vi "Eye Movement Analyser.vi"(7 "Data Output":T12 {"Data Channels" format="%.2f"}) -> ()   [LabVIEW 2016]
uses:
  core/type-defs/TD_Time Series.ctl
  core/type-defs/TD_Impulse Parameter.ctl
  core/private/Impulse Analyser state.ctl
  core/type-defs/TD_Event Sequencer.ctl
  <vilib>/Utility/miscctls.llb/LVRowAndColumnUnsignedTypeDef.ctl
  <vilib>/Analysis/baseanly.llb/Unit Vector (DBL).vi
  <vilib>/Analysis/1siggen.llb/Ramp Pattern by Samples.vi
  <vilib>/Analysis/baseanly.llb/Real Dot Product.vi
  <vilib>/Analysis/baseanly.llb/Mean (DBL).vi
  <vilib>/Utility/inputDevices.llb/mouseAcquire.vi
  <userlib>/_OpenG.lib/comparison/comparison.llb/Boolean Changed__ogtk.vi
  plugins/Mars 3D/Mars3D_autosort.vi
  <vilib>/Utility/file.llb/Read From Spreadsheet File (DBL).vi
  <userlib>/_OpenG.lib/file/file.llb/File Exists - Scalar__ogtk.vi
  <userlib>/_OpenG.lib/array/array.llb/Sort 1D Array (I32)__ogtk.vi
  core/Classes/Graph Manager/Graph Manager.lvclass
  comm/impulse/impulse functions.lvlib
  comm/comm.lvlib
  plugins/Report/generate report.lvlib
  comm/quaternion/quaternion.lvlib
  comm/fick-matrix/fick-matrix.lvlib
  <vilib>/Analysis/NI_AALBase.lvlib
  <vilib>/Analysis/NI_AALPro.lvlib
  <vilib>/Analysis/baseanly.llb/A x Vector.vi
  core/core.lvlib
  comm/double click/double click.lvlib
  plugins/plugin data.lvlib
  <vilib>/ptbypt/NI_PtbyPt.lvlib
  comm/nan operations/nan operations.lvlib
panel:
  out "Time series Trace":cluster{dbl, dbl, dbl[][]}(graph) caption="Waveform Graph"
  in  "Tab Control":T1(tab)
  in  "EyeSeeCam":bool
  in  "Chair":bool
  in  "Mars Training":bool
  in  "3D Chincilla":bool
  in  "Mars 3D 2":bool
  in  "Mars 3D":bool
  in  "JHOC":bool
  in  "Load Data":bool
  in  "Wireless":bool
  in  "Append Data":bool
  in  "Btn Clear Temp LVS":bool
  in  "Update Batch File":bool
  in  "Load Batch File":bool
  in  "Batch Next":bool
  in  "Experiment Files":i32(listbox)
  in  "Parameter Time Series":T2 {"time offset" format="%.3f"; "Gain" format="%.1f"; "Offset" format="%.1f"; "List 1" items=["Hz Position-in-Head", "Hz Velocity-in-Head", "Hy Position-in-Head", "Hy Velocity-in-Head", "Hx Position-in-Head", "Hx Velocity-in-Head", "Hl Velocity-in-Head", "Hr Velocity-in-Head", "Lx Position-in-Head", "Ly Position-in-Head", "Lz Position-in-Head", "Lx Velocity-in-Head", "Ly Velocity-in-Head", "Lz Velocity-in-Head", "Ll Velocity-in-Head", "Lr Velocity-in-Head", "Rx Position-in-Head", "Ry Position-in-Head", "Rz Position-in-Head", "Rx Velocity-in-Head", "Ry Velocity-in-Head", "Rz Velocity-in-Head", "Rl Velocity-in-Head", "Rr Velocity-in-Head", "Target on/off", "aux input 1", "aux input 2", " ", "", "", "", "Target Hor", "Target Ver", ""]}
  in  "Filter Method":u16(ring)=1 items=["Savitzky Golay", "FIR Filter", "Spline"]
  out "Tab Control 2":enum32{"Page 2", "Page 3", "Page 1"}(tab)=enum."Page 3"
  in  "Filter characteristics":T3={"Filter type"=enum."Lowpass", "Order"=50, "Higher pass freq"=40.0, "Lower pass freq"=40.0} {"Lower pass freq" format="%.2f"; "Higher pass freq" format="%.2f"}
  in  "Filter Data":bool
  in  "Gl Spline":bool caption="Enable Spline for all Channels"
  out "R-sq":dbl
  in  "Spline balance parameter":dbl=0.9 min=0.9 max=1.0 step=1e-07 format="%#_7g"
  in  "spline":bool
  in  "Interpolate":bool=TRUE
  in  "S-pline":bool
  out "calibration filename":string
  out "filename":string
  in  "Fixed Time 2":bool caption="Fixed Time"
  in  "Fixed Amplitude 2":bool caption="Fixed Amplitude"
  out "dY":dbl format="%#12.3f"
  out "dX":dbl format="%#10.1f"
  in  "Time Cursor Color 2":u32(colorbox)=16711680
  in  "Time Curser Y2":dbl caption="Y:" format="%_4g"
  in  "Time Curser X2":dbl caption="X:" format="%_4g"
  in  "Time Cursor Color 1":u32(colorbox)=16711680
  in  "Time Curser Y1":dbl caption="Y:" format="%_4g"
  in  "Time Curser X1":dbl caption="X:" format="%_4g"
  in  "Cut":bool
  in  "Keep in range":bool
  in  "Generate New Plot":bool
  out "Impulse Trace":cluster{dbl, dbl, "Impulses":dbl[][]}(graph)
  in  "Asymmetry Plot":bool
  in  "Main Sequence Saccade":bool
  in  "Time Constant Plugin":bool
  in  "Reset to Raw":bool
  in  "Analyze Saccades":bool
  in  "Autosort Name":string
  in  "Auto Sort Parameter":u16(ring) items=["xxx"]
  in  "Impulse Analyser":bool
  in  "Gain and Phase":bool
  in  "Dots":bool
  in  "off and gains perm":bool
  in  "Saccade Velocity":bool
  in  "De-Saccading":bool
  in  "Impulse Parameters":bool
  in  "Group Analyser":bool
  in  "Threshold 2 [% of TH-1]":i32(slide) scale=0.0..100.0
  in  "Tolerance [ms]":dbl(slide)=39.7 step=0.1 scale=0.0..100.0
  in  "Tab Control 3":T4(tab)
  in  "Eye Movement Analyser":bool
  in  "Trigger Method":T5(ring)
  in  "Impulse surround":T6={"Pre Impulse (ms)"=150, "Post Impulse (ms)"=150, "LARP / RALP trigger Vel"=15.0} {"LARP / RALP trigger Vel" format="%.2f"}
  in  "Impulse Characteristics":T7={"Min Vel /Trigger"=90.0, "Width / Offset (ms)"=100, "Maximum Velocity"=300.0} {"Maximum Velocity" format="%.2f"; "Min Vel /Trigger" format="%.2f"}
  in  "Impulse Plane":bool
  in  "Trigger Channel (Other)":u16(ring)=1 items=["Hz Position-in-Head", "Hz Velocity-in-Head", "Hy Position-in-Head", "Hy Velocity-in-Head", "Hx Position-in-Head", "Hx Velocity-in-Head", "Hl Velocity-in-Head", "Hr Velocity-in-Head", "Lx Position-in-Head", "Ly Position-in-Head", "Lz Position-in-Head", "Lx Velocity-in-Head", "Ly Velocity-in-Head", "Lz Velocity-in-Head", "Ll Velocity-in-Head", "Lr Velocity-in-Head", "Rx Position-in-Head", "Ry Position-in-Head", "Rz Position-in-Head", "Rx Velocity-in-Head", "Ry Velocity-in-Head", "Rz Velocity-in-Head", "Rl Velocity-in-Head", "Rr Velocity-in-Head", "Target on/off", "aux input 1", "aux input 2", " ", "", "", "", "Target Hor", "Target Ver", ""]
  in  "Del Autosort":bool
  in  "Add Autosort":bool
  in  "Cross Correlation":bool
  in  "Impulse Characteristic from Cursor":bool caption="Select one periode of the signal"
  in  "Default":bool
  in  "Add Autosort OK":bool
  in  "Add Autosort Cancel":bool
  in  "Accel Threshold [TH-1]":dbl(slide)=3000.0 step=10.0 scale=100.0..1000000.0
  in  "Velocity Threshold":i32(slide)=203 scale=0.0..400.0
  in  "SD for Outlier detection":dbl(slide) scale=0.0..5.0
  in  "Live Update":bool=TRUE
  in  "Reset To default":bool
  in  "Search Window [ms]":i32(slide)=151 scale=0.0..500.0
  in  "Capture Saccade":bool=TRUE
  in  "Display Saccade":bool
  in  "Saccade width [ms]":cluster{i32, i32}(slide)={0, 3} scale=0.0..400.0
  out "Fits a line to a noisy slow-phase. First 3 channels in plot window (above) must be x, y, and z eye position in that order.":dbl[][](graph)
  in  "Sac Vel":bool
  out "HOR\n\nLARP\n\nRALP":dbl[](array[numeric]) format="%#_2g"
  out "X deg/s      Y deg/s      Z deg/s":dbl[](array[numeric]) format="%#_3g"
  out "Mean Ch 1":dbl
  out "Mean Ch2":dbl
  out "Mean Ch3":dbl
  in  "Only Use TH-2":bool
  out "Other Trigger channel":bool
  in  "Shortcut 3":bool
  in  "Shortcut 2":bool
  in  "Shortcut 1":bool
  out "Acc":dbl
  out "Vel.":dbl
  out "Freq.":dbl
  out "Stimulus type":string
  out "No. Imp":i32 caption="# Imp"
  in  "Help":bool
  in  "Options":bool
  in  "Save Image Impulse":bool
  in  "Export TS":bool
  in  "Save Data":bool
  in  "Export Data":bool
  in  "Generate Report":bool
  in  "Redo":bool
  in  "Undo Last":bool
  in  "Undo Last 2":bool
  in  "Tab Control Impuls":enum32{"Page 1", "Page 3", "Page 2"}(tab)
  in  "Parameter Impuls Series":T8 caption="Offset    Gain       Inv                      Channel                            Vis   Sac" {"Gain" format="%.1f"; "Offset" format="%.1f"; "Channel" items=["Hz Position-in-Head", "Hz Velocity-in-Head", "Hy Position-in-Head", "Hy Velocity-in-Head", "Hx Position-in-Head", "Hx Velocity-in-Head", "Hl Velocity-in-Head", "Hr Velocity-in-Head", "Lx Position-in-Head", "Ly Position-in-Head", "Lz Position-in-Head", "Lx Velocity-in-Head", "Ly Velocity-in-Head", "Lz Velocity-in-Head", "Ll Velocity-in-Head", "Lr Velocity-in-Head", "Rx Position-in-Head", "Ry Position-in-Head", "Rz Position-in-Head", "Rx Velocity-in-Head", "Ry Velocity-in-Head", "Rz Velocity-in-Head", "Rl Velocity-in-Head", "Rr Velocity-in-Head", "Target on/off", "aux input 1", "aux input 2", " ", "", "", "", "Target Hor", "Target Ver", ""]}
  in  "Generate New Impulse Plot":bool
  in  "Mean and STD":bool
  in  "Impulse dir":bool
  in  "Impulse Plane 2":T9(ring)=enum."Yaw" caption="Plane"
  in  "Reset Save Options":bool
  in  "Aligning Channel":u16(ring)=5 items=["Hz Position-in-Head", "Hz Velocity-in-Head", "Hy Position-in-Head", "Hy Velocity-in-Head", "Hx Position-in-Head", "Hx Velocity-in-Head", "Hl Velocity-in-Head", "Hr Velocity-in-Head", "Lx Position-in-Head", "Ly Position-in-Head", "Lz Position-in-Head", "Lx Velocity-in-Head", "Ly Velocity-in-Head", "Lz Velocity-in-Head", "Ll Velocity-in-Head", "Lr Velocity-in-Head", "Rx Position-in-Head", "Ry Position-in-Head", "Rz Position-in-Head", "Rx Velocity-in-Head", "Ry Velocity-in-Head", "Rz Velocity-in-Head", "Rl Velocity-in-Head", "Rr Velocity-in-Head", "Target on/off", "aux input 1", "aux input 2", " ", "", "", "", "Target Hor", "Target Ver", ""]
  in  "Horizontal Align":bool
  in  "Vertical Align":bool
  in  "Acceleration":bool
  in  "Autosize Parameter Set":i8(ring) caption="Trigger Set" items=["No Set selected", "Mars 3D", "", "3D Chinchilla", "", "visStim", "", "", "", "", "Human Rotary Chair"]
  in  "Trace":i32 min=0 max=1000
  in  "Paint delete":bool=TRUE
  in  "Cut After":bool
  in  "Cut Before":bool
  in  "Fixed Time":bool
  in  "Fixed Amplitude":bool
  in  "Impuls Cursor Y":dbl caption="Y:"
  in  "Impuls Cursor X":dbl caption="X:"
  out "loaded filename":path
  in  "Head coord":bool
  in  "Target position":T10(ring)
  in  "H":dbl format="%.2f"
  in  "Change coord":bool
  in  "Old Impulse positions for Undo":T11(array[cluster]) {"Amplitude offset" format="%.2f"}
  in  "Impulse Positions":T11(array[cluster]) {"Amplitude offset" format="%.2f"}
  out "axis info":T13
  in  "Delete Impulse":bool
  out "LVS data path":path=path "/Macintosh HD/Users/patrick/Studium/Diploma Thesis/Data Analysis"
  in  "Stop":bool
  in  "Human VOG":bool
  in  "galvanic":bool
  in  "COR":bool
  in  "T":dbl format="%.2f"
  in  "V":dbl format="%.2f"
  in  "Optotrak":bool
  in  "Finnish":bool
  in  "NTA":bool
  in  "ASCII":bool
  in  "Process Coils Data 2":bool
  in  "Process Animal Data":bool
  in  "Process Coils Data":bool
  out "Processing":bool
  # "Description"
  # "<-- Belongs Here"
  # "Rarely used buttons"
  # "FOR COORD\nCHANGE ORDER IS\nXvel,\nYvel,\nZvel,\nLvel,\nRvel"
  # "Cursor:"
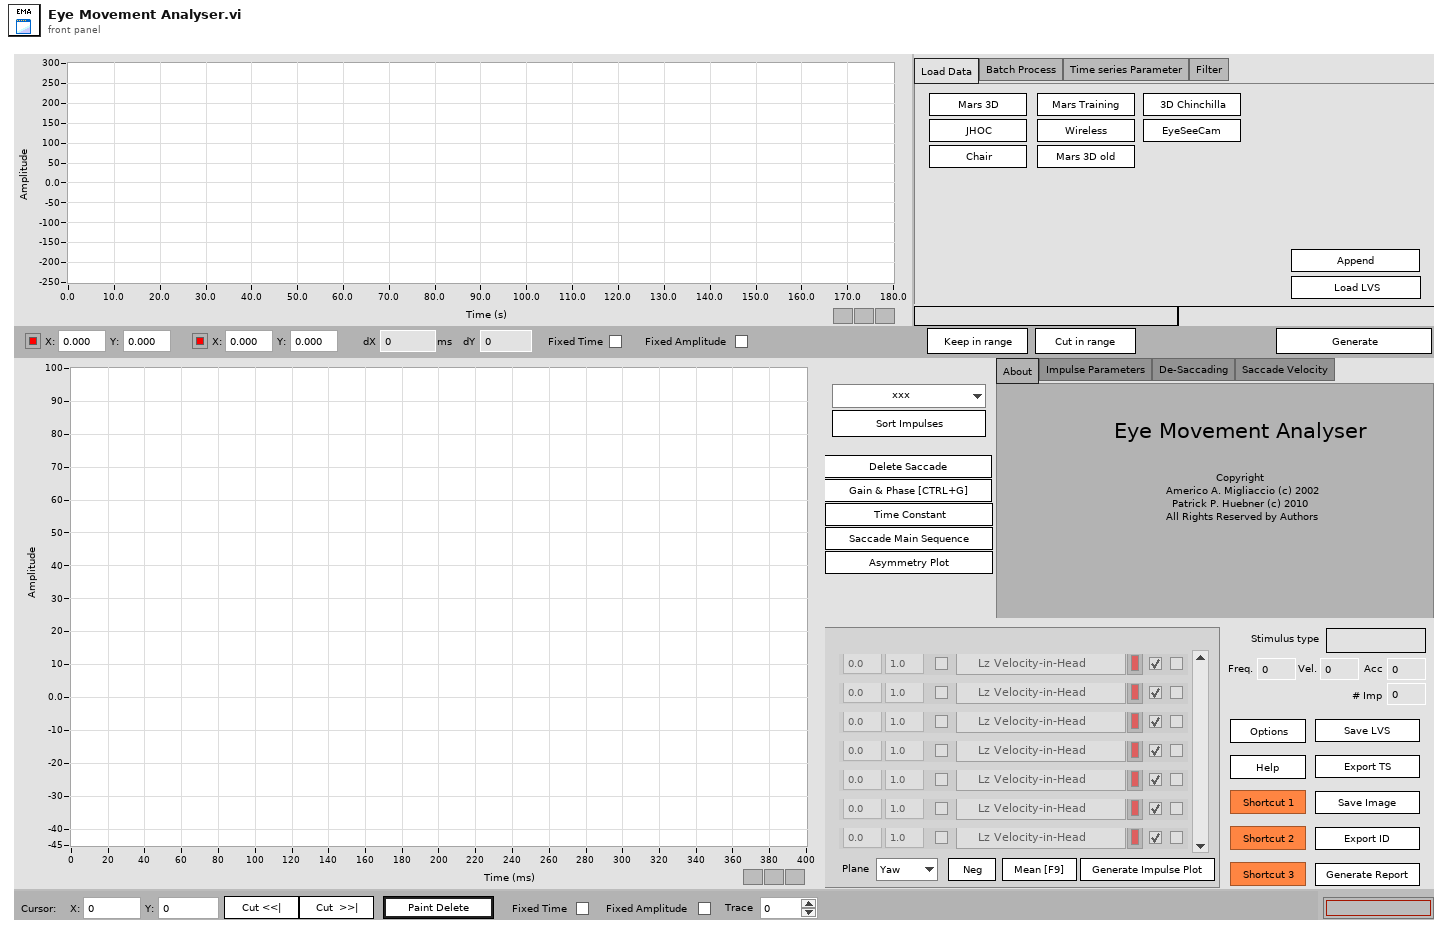
[diagram p1: front panel]
types:
  T1 = enum32{"Load Data", "Batch Process", "Time series Parameter", "Filter"}
  T2 = typedef "core.lvlib/TD_Time Series.ctl" = cluster{"time offset":dbl, "Offset":dbl, "Gain":dbl, "inverse":bool, "filter data":bool, "dots":bool, "interpolate":bool, "List 1":u16, "Color Box":u32, "Boolean":bool}[]
  T3 = cluster{"Filter type":enum32{"Lowpass", "Highpass", "Bandpass", "Bandstop"}, "Order":i32, "Higher pass freq":dbl, "Lower pass freq":dbl}
  T4 = enum32{"About", "Impulse Parameters", "De-Saccading", "Saccade Velocity"}
  T5 = enum16{"Peak Detektion", "Rising Edge", "Falling Edge", "Rising Edge (multiple)", "Falling Edge (multiple)"}
  T6 = cluster{"Pre Impulse (ms)":i32, "Post Impulse (ms)":i32, "LARP / RALP trigger Vel":dbl}
  T7 = cluster{"Min Vel /Trigger":dbl, "Width / Offset (ms)":i32, "Maximum Velocity":dbl}
  T8 = typedef "core.lvlib/TD_Impulse Parameter.ctl" = cluster{"Color":u32, "Visible":bool, "Channel":u16, "Invert":bool, "Desaccade":bool, "Offset":dbl, "Gain":dbl}[]
  T9 = enum16{"Other", "Yaw", "Pitch", "Roll", "LARP", "RALP"}
  T10 = enum16{"Far 0", "Far Left 20", "Far Left 30", "Far right 30", "Far Right 20", "Near 0", "Near Left 20", "Near Right 20"}
  T11 = cluster{"Start":i32, "End":i32, "Impulse Plane":enum16{"Other", "Yaw", "Pitch", "Roll", "LARP", "RALP"}, "Impulse Direction +ve?":bool, "Time offset":i32, "Amplitude offset":dbl}[]
  T12 = cluster{"Data Channels":dbl[][], "Sample Rate":i32, "Channel List":string[]}
  T13 = cluster{"Horizontal":i32, "Vertical":i32, "Scrolling":i32}
  T14 = typedef "Impulse Analyser state.ctl" = enum16{"--- System ---", "Panel Monitoring", "Check Save Status", "Initialize", "Initialise GUI", "Quit", "--- Import ---", "Desaccade Time Data", "Desaccade Time Data Background", "Paint Delete", "Load Batch Log File", "Make Batch List", "Update Batch List", "Delete Batch List", "Delete Temporary LVS", "Save Temporary LVS", "Check for Batch LVS", "Process 3D Chinchilla", "Find default parameter", "Mars3D old", "Chair", "EyeSeeCam", "Open last session", "Save RAW", "Auto Impulse Parameter", "Save Image", "Wireless", "Process Coils Data", "Process JHOC Data", "Process Animal Data", "Australian Data", "ASCII", "Mars 3D", "Mars 3D Training", "Position Mean Plugin", "plot generator plugin", "Human VOG system", "Optotrak", "spline", "COR", "galvanic", "Generate New Time Plot", "Make off and gains permanent", "Generate New Impulse Plot", "Defer Impulse Plot", "Fill Impulse Plot Data", "Scale Impulse Plot", "Un-Defer Impulse Plot", "Snap Impulse Cursor", "Extract Saccades", "Impulse Analyser", "NTA", "Acceleration", "Saccade Velocity", "Horizontal Align", "Vertical Align", "Delete Impulse", "Cut Before", "Cut After", "Filter Data", "Undo Last", "Redo", "Mean and STD", "Group Analyser", "Generate Report", "Phase Plots", "Gain and Phase", "Example Plugin", "Time Constant Plugin", "Export Data", "Export Time Series Data", "Append Data", "Save Data", "Load Data", "Cut in Range", "Keep in range", "Stop"}
  T15 = typedef "TD_Event Sequencer.ctl" = enum16{"Core", "Plugins"}
  T16 = enum8{"Enabled", "Disabled", "Disabled and Grayed Out"}
  T17 = cluster{"Save RAW":bool, "Save Options":bool, "Save IMAGE":bool, "Cycle Nr for Saccades":cluster{"POS":i32, "NEG":i32}, "Paint Delete":bool, "device ID":refnum<k1>, "Delete-Array":i32[], "Double Click":refnum<event-registration>, "DC file":path, "Session saved?":bool}
  T18 = cluster{"Start":i32, "End":i32, "Impulse Plane":enum16{"Other", "Yaw", "Pitch", "Roll", "LARP", "RALP"}, "Impulse Direction +ve?":bool, "Time offset":i32, "Amplitude offset":dbl}
  T19 = enum16{"open", "open or create", "create or replace", "create", "open (read only)"}
  T20 = typedef "LVRowAndColumnUnsignedTypeDef.ctl" = cluster{"Row":u32, "Column":u32}
  T21 = enum16{"open", "replace", "create", "open or create", "replace or create", "replace or create with confirmation"}
  T22 = enum16{"Left Button", "Center Button", "Right Button", "Window Close"}
  T23 = cluster{"Impulse Positions":cluster{"Start":i32, "End":i32, "Impulse Plane":enum16{"Other", "Yaw", "Pitch", "Roll", "LARP", "RALP"}, "Impulse Direction +ve?":bool, "Time offset":i32, "Amplitude offset":dbl}[], "Old Impulse positions for Undo":cluster{"Start":i32, "End":i32, "Impulse Plane":enum16{"Other", "Yaw", "Pitch", "Roll", "LARP", "RALP"}, "Impulse Direction +ve?":bool, "Time offset":i32, "Amplitude offset":dbl}[], "No. Imp":i32, "Parameter Time Series":T2, "Parameter Impuls Series":T8, "Experiment Parameters":cluster{"Freq":dbl, "Vel":i32, "Acc":i32, "Stimulus":string}, "Autosort File":refnum<file>, "Data File":cluster{"Data Channels":dbl[][], "Sample Rate":i32, "Channel List":string[]}, "Experiment data path":path, "Image data path":path, "LVS data path":path, "Raw copy path":path, "filename":string, "desaccading parameters":cluster{"Tolerance":i32, "Acc Range":dbl, "Sample Rate":i32, "Impulse Plane 2":enum16{"Other", "Yaw", "Pitch", "Roll", "LARP", "RALP"}, "Impulse dir":bool}, "Experiment Parameters 2":cluster{"Subject":string, "Strain":string, "Rotation plane":string, "Experimenter":string, "Trial":dbl, "Time":dbl}, "Excel":cluster{"Excel._Application":refnum<k7>, "Use Excel":bool, "Worksheet SINE":refnum<k7>, "Row SINE":i32, "Worksheet TRANS":refnum<k7>, "Row TRANS":i32}, "Session Config File":refnum<file>, "Autosort Parameter Set":i32, "EMA Version":string, "desacc ":cluster{"Threshold 1 [Acc]":dbl, "Threshold 2 [% of TH1]":i32, "tolerance":i32, "Search WD ":dbl, " always use TH2":bool, "Range":dbl, "Max time":dbl, "Min time":dbl}}
  T24 = cluster{"Subject":string, "Strain":string, "Rotation plane":string, "Experimenter":string, "Trial":dbl, "Time":dbl}
  T25 = cluster{"Freq":dbl, "Vel":i32, "Acc":i32, "Stimulus":string}
  T26 = cluster{"Impulse Positions":cluster{"Start":i32, "End":i32, "Impulse Plane":enum16{"Other", "Yaw", "Pitch", "Roll", "LARP", "RALP"}, "Impulse Direction +ve?":bool, "Time offset":i32, "Amplitude offset":dbl}[], "Old Impulse positions for Undo":cluster{"Start":i32, "End":i32, "Impulse Plane":enum16{"Other", "Yaw", "Pitch", "Roll", "LARP", "RALP"}, "Impulse Direction +ve?":bool, "Time offset":i32, "Amplitude offset":dbl}[], "No. Imp":i32}
  T27 = typedef "LVPoint32TypeDef.ctl" = cluster{"Horizontal":i32, "Vertical":i32}
  T28 = cluster{"button 1":bool, "button 2":bool, "button 3":bool, "button 4":bool}
  T29 = cluster{"Fixed Time":bool, "Fixed Amplitude":bool}
  T30 = typedef "core.lvlib/TD_Statemachine-Data.ctl" = cluster{"Impulse Positions":cluster{"Start":i32, "End":i32, "Impulse Plane":enum16{"Other", "Yaw", "Pitch", "Roll", "LARP", "RALP"}, "Impulse Direction +ve?":bool, "Time offset":i32, "Amplitude offset":dbl}[], "Old Impulse positions for Undo":cluster{"Start":i32, "End":i32, "Impulse Plane":enum16{"Other", "Yaw", "Pitch", "Roll", "LARP", "RALP"}, "Impulse Direction +ve?":bool, "Time offset":i32, "Amplitude offset":dbl}[][], "No. Imp":i32, "Parameter Time Series":T2, "Parameter Impuls Series":T8, "Experiment Parameters":cluster{"Freq":dbl, "Vel":i32, "Acc":i32, "Stimulus":string}, "Autosort File":refnum<file>, "Data File":cluster{"Data Channels":dbl[][], "Sample Rate":i32, "Channel List":string[]}, "Experiment data path":path, "Image data path":path, "LVS data path":path, "Raw copy path":path, "filename":string, "desaccading parameters":cluster{"Tolerance":i32, "Acc Range":dbl, "Sample Rate":i32, "Impulse Plane 2":enum16{"Other", "Yaw", "Pitch", "Roll", "LARP", "RALP"}, "Impulse dir":bool}, "Experiment Parameters 2":cluster{"Subject":string, "Strain":string, "Rotation plane":string, "Experimenter":string, "Trial":dbl, "Time":dbl}, "Excel":cluster{"Excel._Application":refnum<k7>, "Use Excel":bool, "Worksheet SINE":refnum<k7>, "Row SINE":i32, "Worksheet TRANS":refnum<k7>, "Row TRANS":i32}, "Session Config File":refnum<file>, "Autosort Parameter Set":i32, "EMA Version":string, "desacc ":cluster{"Threshold 1 [Acc]":dbl, "Threshold 2 [% of TH1]":i32, "tolerance":i32, "Search WD ":dbl, " always use TH2":bool, "Range":dbl, "Max time":dbl, "Min time":dbl, "Velocity Threshold":i32}, "Cycle Nr for Saccades":cluster{"POS":i32, "NEG":i32}, "Undo Counter":i32, "History Length":i32, "Redo Counter":i32, "Histpry Position":i32, "Raw Data File":cluster{"Data Channels":dbl[][], "Sample Rate":i32, "Channel List":string[]}, "calibration name":string}
  T31 = cluster{"Threshold 1 [Acc]":dbl, "Threshold 2 [% of TH1]":i32, "tolerance":i32, "Search WD ":dbl, " always use TH2":bool, "Range":dbl, "Max time":dbl, "Min time":dbl, "Velocity Threshold":i32}
  T32 = cluster{"Tolerance [ms]":dbl, "Accel Threshold [TH-1]":dbl, "Sample Rate":i32, "Impulse Plane 2":enum16{"Other", "Yaw", "Pitch", "Roll", "LARP", "RALP"}, "Impulse dir":bool}
  T33 = typedef "eventvkey.ctl" = enum16{"ASCII", "Enter", "Return", "Shift", "Ctrl", "Alt", "Cmd", "Opt", "Caps", "NumLock", "Clear", "Break", "Up", "Down", "Left", "Right", "Insert", "Delete", "Home", "End", "PageUp", "PageDown", "Escape", "Help", "Pause", "ScrollLock", "F1", "F2", "F3", "F4", "F5", "F6", "F7", "F8", "F9", "F10", "F11", "F12", "F13", "F14", "F15", "F16", "F17", "F18", "F19", "F20", "F21", "F22", "F23", "F24", "Play", "VolumeUp", "VolumeDown", "Mute", "Two Byte Char"}
  T34 = cluster{"Shift":bool, "Ctrl":bool, "Alt":bool, "Cmd":bool, "Opt":bool}
  T35 = cluster{"Start":i32, "End":i32, "Impulse Plane":enum16{"Other", "Yaw", "Pitch", "Roll", "LARP", "RALP"}, "Impulse Direction +ve?":bool, "Time offset":i32, "Amplitude offset":dbl}[][]
  T36 = enum32{"invalid app kind", "Development System", "Run Time System", "Student Edition", "Embedded LabVIEW", "Evaluation", "Custom"}
  T37 = cluster{"Tolerance":i32, "Acc Range":dbl, "Sample Rate":i32, "Impulse Plane 2":enum16{"Other", "Yaw", "Pitch", "Roll", "LARP", "RALP"}, "Impulse dir":bool}
  T38 = cluster{"Impulse Positions":cluster{"Start":i32, "End":i32, "Impulse Plane":enum16{"Other", "Yaw", "Pitch", "Roll", "LARP", "RALP"}, "Impulse Direction +ve?":bool, "Time offset":i32, "Amplitude offset":dbl}[], "Old Impulse positions for Undo":cluster{"Start":i32, "End":i32, "Impulse Plane":enum16{"Other", "Yaw", "Pitch", "Roll", "LARP", "RALP"}, "Impulse Direction +ve?":bool, "Time offset":i32, "Amplitude offset":dbl}[][], "No. Imp":i32, "Parameter Time Series":T2, "Parameter Impuls Series":T8, "Experiment Parameters":cluster{"Freq":dbl, "Vel":i32, "Acc":i32, "Stimulus":string}, "Data File":cluster{"Data Channels":dbl[][], "Sample Rate":i32, "Channel List":string[]}, "Experiment data path":path, "Image data path":path, "LVS data path":path, "Raw copy path":path, "filename":string, "desaccading parameters":cluster{"Tolerance":i32, "Acc Range":dbl, "Sample Rate":i32, "Impulse Plane 2":enum16{"Other", "Yaw", "Pitch", "Roll", "LARP", "RALP"}, "Impulse dir":bool}, "Experiment Parameters 2":cluster{"Subject":string, "Strain":string, "Rotation plane":string, "Experimenter":string, "Trial":dbl, "Time":dbl}, "Autosort Parameter Set":i32, "calibration name":string}
  T39 = cluster{"Data Output":cluster{"Data Channels":dbl[][], "Sample Rate":i32, "Channel List":string[]}, "Data OUT":T30}
  T40 = cluster{"Autosize Parameter Set 2":cluster{"Trigger Ch":i32, "Min Vel":dbl, "MaxVel":dbl, "Width":i32, "Pre Impuls":i32, "Post Impuls":i32, "Pitch":dbl, "Name":string, "Other Trigger":bool, "Cross Corr":bool, "Default":cluster{"Freq":dbl, "Vel":dbl, "Acc":dbl, "Stimulus":string}}[]}[]
  T41 = cluster{"Autosize Parameter Set 2":cluster{"Trigger Ch":i32, "Min Vel":dbl, "MaxVel":dbl, "Width":i32, "Pre Impuls":i32, "Post Impuls":i32, "Pitch":dbl, "Name":string, "Other Trigger":bool, "Cross Corr":bool, "Default":cluster{"Freq":dbl, "Vel":dbl, "Acc":dbl, "Stimulus":string}}[]}
  T42 = cluster{"Trigger Ch":i32, "Min Vel":dbl, "MaxVel":dbl, "Width":i32, "Pre Impuls":i32, "Post Impuls":i32, "Pitch":dbl, "Name":string, "Other Trigger":bool, "Cross Corr":bool, "Default":cluster{"Freq":dbl, "Vel":dbl, "Acc":dbl, "Stimulus":string}}[]
  T43 = cluster{"Freq":dbl, "Vel":dbl, "Acc":dbl, "Stimulus":string}
  T44 = cluster{"Freq":bool, "Vel":bool, "Acc":bool, "Stimulus":bool}
  T45 = cluster{"Trigger Ch":i32, "Min Vel":dbl, "MaxVel":dbl, "Width":i32, "Pre Impuls":i32, "Post Impuls":i32, "Pitch":dbl, "Name":string, "Other Trigger":bool, "Cross Corr":bool, "Default":cluster{"Freq":dbl, "Vel":dbl, "Acc":dbl, "Stimulus":string}}
  T46 = typedef "imagedata.ctl" = cluster{"image type":i32, "image depth":i32, "image":u8[], "mask":u8[], "colors":u32[], "Rectangle":cluster{"left":i16, "top":i16, "right":i16, "bottom":i16}}
  T47 = typedef "plugin data.lvlib/Plugin Shared Data.ctl" = cluster{"Impulse Positions":cluster{"Start":i32, "End":i32, "Impulse Plane":enum16{"Other", "Yaw", "Pitch", "Roll", "LARP", "RALP"}, "Impulse Direction +ve?":bool, "Time offset":i32, "Amplitude offset":dbl}[], "Parameter Impuls Series":T8, "Data File":cluster{"Data Channels":dbl[][], "Sample Rate":i32, "Channel List":string[]}, "desacc ":cluster{"Threshold 1 [Acc]":dbl, "Threshold 2 [% of TH1]":i32, "tolerance":i32, "Search WD ":dbl, " always use TH2":bool, "Range":dbl, "Max time":dbl, "Min time":dbl, "Velocity Threshold":i32}, "Experiment Parameters 2":cluster{"Subject":string, "Strain":string, "Rotation plane":string, "Experimenter":string, "Trial":dbl, "Time":dbl}}
  T48 = typedef "TC_Plugin.lvlibp/plugin data.lvlib/Plugin Shared Data.ctl" = cluster{"Impulse Positions":cluster{"Start":i32, "End":i32, "Impulse Plane":enum16{"Other", "Yaw", "Pitch", "Roll", "LARP", "RALP"}, "Impulse Direction +ve?":bool, "Time offset":i32, "Amplitude offset":dbl}[], "Parameter Impuls Series":T49, "Data File":cluster{"Data Channels":dbl[][], "Sample Rate":i32, "Channel List":string[]}, "desacc ":cluster{"Threshold 1 [Acc]":dbl, "Threshold 2 [% of TH1]":i32, "tolerance":i32, "Search WD ":dbl, " always use TH2":bool, "Range":dbl, "Max time":dbl, "Min time":dbl, "Velocity Threshold":i32}, "Experiment Parameters 2":cluster{"Subject":string, "Strain":string, "Rotation plane":string, "Experimenter":string, "Trial":dbl, "Time":dbl}}
  T49 = typedef "comm.lvlibp/TD_Impulse Parameter.ctl" = cluster{"Color Box":u32, "Boolean":bool, "List 2":u16, "Boolean 2":bool, "Boolean 3":bool, "Offset":dbl, "Gain":dbl}[]
  T50 = cluster{"Data Output":cluster{"Data Channels":dbl[][], "Sample Rate":i32, "Channel List":string[]}, "output cluster":cluster{"Impulse Positions":cluster{"Start":i32, "End":i32, "Impulse Plane":enum16{"Other", "Yaw", "Pitch", "Roll", "LARP", "RALP"}, "Impulse Direction +ve?":bool, "Time offset":i32, "Amplitude offset":dbl}[], "Old Impulse positions for Undo":cluster{"Start":i32, "End":i32, "Impulse Plane":enum16{"Other", "Yaw", "Pitch", "Roll", "LARP", "RALP"}, "Impulse Direction +ve?":bool, "Time offset":i32, "Amplitude offset":dbl}[], "No. Imp":i32, "Parameter Time Series":T2, "Parameter Impuls Series":T8, "Experiment Parameters":cluster{"Freq":dbl, "Vel":i32, "Acc":i32, "Stimulus":string}, "Autosort File":refnum<file>, "Data File":cluster{"Data Channels":dbl[][], "Sample Rate":i32, "Channel List":string[]}, "Experiment data path":path, "Image data path":path, "LVS data path":path, "Raw copy path":path, "filename":string, "desaccading parameters":cluster{"Tolerance":i32, "Acc Range":dbl, "Sample Rate":i32, "Impulse Plane 2":enum16{"Other", "Yaw", "Pitch", "Roll", "LARP", "RALP"}, "Impulse dir":bool}, "Experiment Parameters 2":cluster{"Subject":string, "Strain":string, "Rotation plane":string, "Experimenter":string, "Trial":dbl, "Time":dbl}, "Excel":cluster{"Excel._Application":refnum<k7>, "Use Excel":bool, "Worksheet SINE":refnum<k7>, "Row SINE":i32, "Worksheet TRANS":refnum<k7>, "Row TRANS":i32}, "Session Config File":refnum<file>, "Autosort Parameter Set":i32, "EMA Version":string, "desacc ":cluster{"Threshold 1 [Acc]":dbl, "Threshold 2 [% of TH1]":i32, "tolerance":i32, "Search WD ":dbl, " always use TH2":bool, "Range":dbl, "Max time":dbl, "Min time":dbl}}}
  T51 = cluster{"Data Output":cluster{"Data Channels":dbl[][], "Sample Rate":i32, "Channel List":string[]}, "output cluster":cluster{"Impulse Positions":cluster{"Start":i32, "End":i32, "Impulse Plane":enum16{"Other", "Yaw", "Pitch", "Roll", "LARP", "RALP"}, "Impulse Direction +ve?":bool, "Time offset":i32, "Amplitude offset":dbl}[], "Old Impulse positions for Undo":cluster{"Start":i32, "End":i32, "Impulse Plane":enum16{"Other", "Yaw", "Pitch", "Roll", "LARP", "RALP"}, "Impulse Direction +ve?":bool, "Time offset":i32, "Amplitude offset":dbl}[], "No. Imp":i32}}
  T52 = enum32{"Lowpass", "Highpass", "Bandpass", "Bandstop"}
  T53 = cluster{dbl, dbl, "Best Cubic Spline Fit":dbl[][]}
  T54 = enum32{"existing file", "new file", "new or existing file", "existing dir", "new dir", "new or existing dir", "existing file (use LLBs)", "new file (use LLBs)", "new or existing file (use LLBs)", "new or existing file or directory (use LLBs)"}
  T55 = cluster{"Color":u32, "Visible":bool, "Channel":u16, "Invert":bool, "Desaccade":bool, "Offset":dbl, "Gain":dbl}
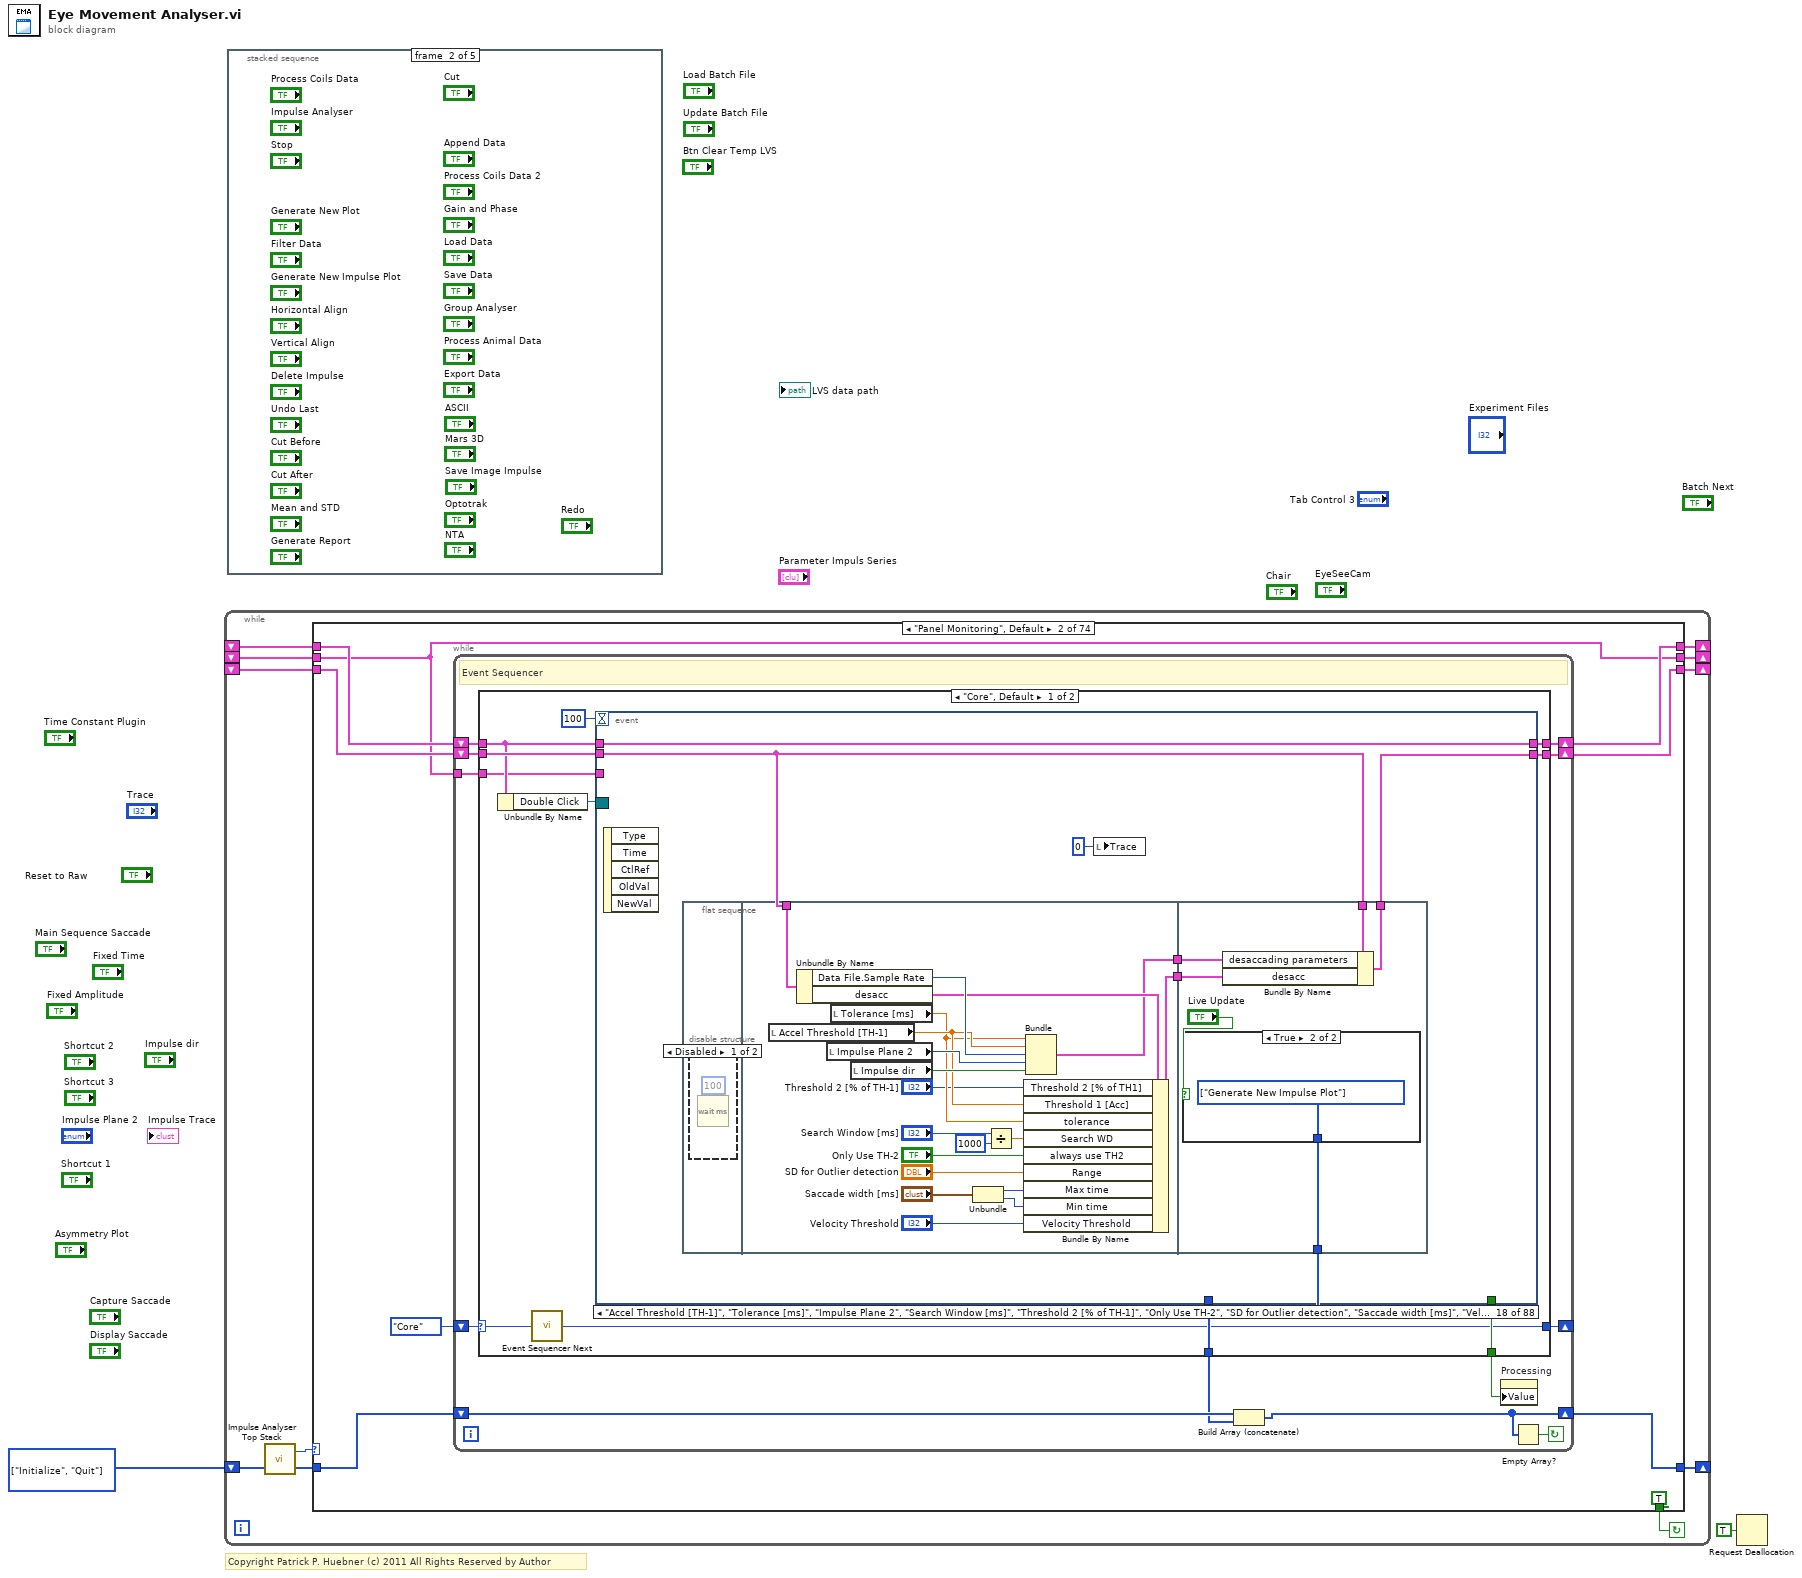
[diagram p0: block diagram]
diagram:
  w1 = T14[] [enum."Initialize", enum."Quit"] items=["--- System ---", "Panel Monitoring", "Check Save Status", "Initialize", "Initialise GUI", "Quit", "--- Import ---", "Desaccade Time Data", "Desaccade Time Data Background", "Paint Delete", "Load Batch Log File", "Make Batch List", "Update Batch List", "Delete Batch List", "Delete Temporary LVS", "Save Temporary LVS", "Check for Batch LVS", "Process 3D Chinchilla", "Find default parameter", "Mars3D old", "Chair", "EyeSeeCam", "Open last session", "Save RAW", "Auto Impulse Parameter", "Save Image", "Wireless", "Process Coils Data", "Process JHOC Data", "Process Animal Data", "Australian Data", "ASCII", "Mars 3D", "Mars 3D Training", "Position Mean Plugin", "plot generator plugin", "Human VOG system", "Optotrak", "spline", "COR", "galvanic", "Generate New Time Plot", "Make off and gains permanent", "Generate New Impulse Plot", "Defer Impulse Plot", "Fill Impulse Plot Data", "Scale Impulse Plot", "Un-Defer Impulse Plot", "Snap Impulse Cursor", "Extract Saccades", "Impulse Analyser", "NTA", "Acceleration", "Saccade Velocity", "Horizontal Align", "Vertical Align", "Delete Impulse", "Cut Before", "Cut After", "Filter Data", "Undo Last", "Redo", "Mean and STD", "Group Analyser", "Generate Report", "Phase Plots", "Gain and Phase", "Example Plugin", "Time Constant Plugin", "Export Data", "Export Time Series Data", "Append Data", "Save Data", "Load Data", "Cut in Range", "Keep in range", "Stop"] ("State stack IN")
  # "Copyright Patrick P. Huebner (c) 2011 All Rights Reserved by Author"
  n1 = while {
    shift-left: _ -> [w11]
    shift-right: [w12] -> _
    shift-right: [w7] -> _
    shift-left: w1 -> [w8]
    shift-right: [w5] -> _
    shift-left: _ -> [w6]
    shift-right: [w4] -> _
    shift-left: _ -> [w3]
    stop <- w13 continue-if-true
    n2 = call "Impulse Analyser Top Stack.vi"("State stack IN"=w8) -> ("State stack OUT"=w9:T14[], "State"=w10:T14)  [unwired: 1 in]
    n3 = case shown="\"Panel Monitoring\", Default" w10 {
      tunnel: w9 -> [w16 w27 _ w694 w707 w732 w737 _ w987 _ w1059 w1079 w1138 w1180 w1200 w1268 w1287 _ _ w1371 _ w1396 w1401 w1406 w1415 w1438 _ w1495 w1507 _ _ _ _ _ w1671 _ w1714 w1731 w1762 w1770 w1801 w1845 w1867 w1875 w1913 w1921 w2056 w2069 _ w2096 w2101 w2109 w2113 w2176 w2215 w2220 _ w2316 w2416 w2461 w2479 w2503 w2533 w2548 w2562 w2598 w2640 w2679 w2703 w2725 w2835 w2879 w2971 w3028]
      tunnel: [TRUE TRUE TRUE TRUE FALSE FALSE TRUE TRUE TRUE TRUE TRUE TRUE TRUE TRUE TRUE TRUE TRUE TRUE TRUE TRUE TRUE TRUE TRUE TRUE TRUE TRUE TRUE TRUE TRUE TRUE TRUE TRUE TRUE TRUE TRUE TRUE TRUE TRUE TRUE TRUE TRUE TRUE TRUE TRUE TRUE TRUE TRUE TRUE TRUE TRUE TRUE TRUE TRUE TRUE TRUE TRUE TRUE TRUE TRUE TRUE TRUE TRUE TRUE TRUE TRUE TRUE TRUE TRUE TRUE TRUE TRUE TRUE TRUE TRUE] -> w13
      tunnel: [w17 w24 w658 w695 w706 w733 w738 w751 w970 w1042 w1062 w1077 w1136 w1186 w1205 w1246 w1288 w1326 w1346 w1372 w1376 w1397 w1402 w1409 w1417 w1433 w1449 w1496 w1548 w1565 w1587 w1613 w1631 w1649 w1665 w1703 w1715 w1752 w1763 w1774 w1786 w1852 w1868 w1872 w1908 w1920 w2057 w2063 w2080 w2091 w2104 w2106 w2114 w2179 w2216 w2225 w2238 w2306 w2438 w2467 w2485 w2510 w2539 w2554 w2560 w2596 w2645 w2680 w2699 w2720 w2836 w2880 w2972 w3024] -> w12
      tunnel: w11 -> [w17 w25 _ w695 w706 w733 w738 w752 w970 w1041 w1062 w1077 w1136 w1186 w1205 w1247 w1288 w1327 w1347 w1372 w1380 w1397 w1402 w1409 w1417 w1434 w1445 w1496 w1548 w1573 w1591 w1612 w1636 w1651 w1666 w1696 w1715 w1720 w1763 w1774 w1785 w1852 w1868 w1872 w1912 w1920 w2058 w2064 w2077 w2087 w2104 w2106 w2114 w2179 w2216 w2225 w2238 w2311 w2420 w2458 w2476 w2506 w2530 w2545 w2561 w2597 w2637 w2677 w2700 w2720 w2836 w2880 w2972 w3024]
      tunnel: [w16 w21 w672 w694 w707 w732 w737 w750 w987 w1040 w1059 w1079 w1138 w1180 w1199 w1268 w1287 w1325 w1344 w1371 w1377 w1396 w1401 w1406 w1415 w1438 w1446 w1495 w1507 w1571 w1595 w1617 w1634 w1654 w1671 w1691 w1714 w1731 w1761 w1770 w1801 w1845 w1867 w1875 w1913 w1921 w2056 w2069 w2074 w2096 w2101 w2109 w2113 w2176 w2215 w2221 w2256 w2316 w2416 w2461 w2479 w2503 w2533 w2548 w2562 w2598 w2640 w2679 w2703 w2725 w2835 w2879 w2971 w3029] -> w7
      tunnel: w6 -> [w18 w23 _ w696 w705 w731 w739 w749 w988 w1044 w1067 w1080 w1139 w1188 w1194 w1228 w1286 w1324 w1343 w1370 w1375 w1395 w1400 w1405 w1414 w1437 w1450 w1494 w1506 w1568 w1594 w1616 w1632 w1650 w1670 w1704 w1713 w1722 w1767 w1776 w1803 w1854 w1870 w1877 w1910 w1919 w2055 w2068 w2084 w2095 w2099 w2108 w2112 w2175 w2214 w2222 w2255 w2309 w2415 w2460 w2478 w2508 w2532 w2547 w2559 w2594 w2634 w2678 w2702 w2723 w2834 w2878 w2970 w3027]
      tunnel: [w18 w22 w667 w696 w705 w731 w739 w748 w988 w1044 w1067 w1080 w1139 w1188 w1194 w1228 w1286 w1324 w1343 w1370 w1375 w1395 w1400 w1405 w1414 w1437 w1450 w1494 w1506 w1567 w1593 w1615 w1632 w1650 w1670 w1704 w1713 w1722 w1766 w1776 w1803 w1854 w1870 w1877 w1910 w1919 w2054 w2062 w2079 w2090 w2099 w2108 w2112 w2175 w2214 w2222 w2254 w2308 w2415 w2460 w2478 w2508 w2532 w2547 w2559 w2594 w2634 w2678 w2702 w2722 w2834 w2878 w2970 w3026] -> w5
      tunnel: [w14 w19 w658 w684 w703 w730 w735 w743 w982 w1043 w1066 w1071 w1130 w1187 w1193 w1227 w1285 w1314 w1342 w1367 w1376 w1394 w1399 w1404 w1411 w1432 w1447 w1493 w1505 w1565 w1587 w1613 w1631 w1649 w1663 w1687 w1711 w1717 w1764 w1775 w1802 w1853 w1869 w1876 w1909 w1918 w2052 w2061 w2076 w2088 w2098 w2107 w2111 w2173 w2213 w2218 w2244 w2306 w2414 w2456 w2474 w2504 w2528 w2543 w2558 w2593 w2632 w2670 w2699 w2719 w2833 w2877 w2969 w3025] -> w4
      tunnel: w3 -> [w14 w19 _ w684 w703 w730 w735 w743 w982 w1043 w1066 w1071 w1130 w1187 w1193 w1227 w1285 w1314 w1342 w1368 _ w1394 w1399 w1404 w1412 w1432 w1447 w1493 w1505 _ _ _ _ _ w1663 w1687 w1712 w1717 w1764 w1775 w1802 w1853 w1869 w1876 w1909 w1918 w2052 w2061 w2076 w2088 w2098 w2107 w2111 w2174 w2213 w2218 w2244 _ w2414 w2456 w2474 w2504 w2528 w2543 w2558 w2593 w2632 w2670 _ w2719 w2833 w2877 w2969 w3025]
      frame "--- System ---" {
      }
      frame "Panel Monitoring", Default {
        n4 = while {
          shift-right: [w36] -> w22
          shift-left: w23 -> [w37]
          shift-right: [w38] -> w24
          shift-left: w25 -> [w39]
          shift-right: [w32] -> w21
          shift-left: w27 -> [w35]
          shift-right: [w30] -> _
          shift-left: TD_Event_Sequencer."Core" ("Enum in") -> [w31]
          tunnel: w19 -> [w28]
          stop <- w33 continue-if-true
          # "Event Sequencer"
          n5 = case shown="\"Core\", Default" w31 {
            selector: w31 -> [w41 w626]
            tunnel: w39 -> [w50 w621]
            tunnel: [w49 w622] -> w38
            tunnel: w37 -> [w48 w624]
            tunnel: [w47 w623] -> w36
            tunnel: [w45 w618] -> w29
            tunnel: [w43 w619] -> w34
            tunnel: [w42 w625] -> w30
            tunnel: w28 -> [w40 _]
            frame "Core", Default {
              n6 = Unbundle By Name(w48) -> ("Double Click"=w44:refnum<event-registration>)
              n7 = call "Event Sequencer Next.vi"("Enum in"=w41) -> ("Enum out"=w42:T15)
              n8 = event shown="[17] \"Accel Threshold [TH-1]\", \"Tolerance [ms]\", \"Impulse Plane 2\", \"Search Window [ms]\", \"Threshold 2 [% of TH-1]\", \"Only Use TH-2\", \"SD for Outlier detection\", \"Saccade width [ms]\", \"Velocity Threshold\", \"Impulse dir\": Value Change" {
                selector: w44 -> [_ _ _ _ _ _ _ _ _ _ _ _ _ _ _ _ _ _ _ _ _ _ _ _ _ _ _ _ _ _ _ _ _ _ _ _ _ _ _ _ _ _ _ _ _ _ _ _ _ _ _ _ _ _ _ _ _ _ _ _ _ _ _ _ _ _ _ _ _ _ _ _ _ _ _ _ _ _ _ _ _ _ _ _ _ _ _ _]
                dyn-events: _ -> [_ _ _ _ _ _ _ _ _ _ _ _ _ _ _ _ _ _ _ _ _ _ _ _ _ _ _ _ _ _ _ _ _ _ _ _ _ _ _ _ _ _ _ _ _ _ _ _ _ _ _ _ _ _ _ _ _ _ _ _ _ _ _ _ _ _ _ _ _ _ _ _ _ _ _ _ _ _ _ _ _ _ _ _ _ _ _ _]
                timeout: 100 -> [_ _ _ _ _ _ _ _ _ _ _ _ _ _ _ _ _ _ _ _ _ _ _ _ _ _ _ _ _ _ _ _ _ _ _ _ _ _ _ _ _ _ _ _ _ _ _ _ _ _ _ _ _ _ _ _ _ _ _ _ _ _ _ _ _ _ _ _ _ _ _ _ _ _ _ _ _ _ _ _ _ _ _ _ _ _ _ _]
                tunnel: w50 -> [w78 w88 w95 w100 w102 w107 w109 w130 w142 w146 w152 w153 w160 w163 w166 w190 w212 w214 w248 _ w254 w260 w268 w274 w281 w284 w290 w293 w296 w300 w303 w310 w315 w318 w322 w324 w333 w363 w373 w386 w392 w399 w404 w407 w410 w413 w416 w425 w479 w497 w500 w503 w506 w507 w513 w518 w523 w527 w530 w533 w536 w539 w542 w545 w548 w551 w554 w557 w560 w563 w566 w569 w572 w575 w578 w581 w584 w587 w590 w593 w596 w599 w602 w605 w608 w611 w614 w617]
                tunnel: [w78 w88 w95 w100 w102 w107 w109 w130 w142 w146 w152 w156 w159 w163 w166 w190 w212 w215 w248 w253 w254 w260 w268 w274 w281 w284 w289 w293 w296 w300 w303 w310 w315 w318 w322 w324 w333 w363 w373 w386 w392 w399 w404 w407 w410 w413 w416 w425 w479 w497 w500 w503 w506 w507 w512 w517 w522 w527 w530 w533 w536 w539 w542 w545 w548 w551 w554 w557 w560 w563 w566 w569 w572 w575 w578 w581 w584 w587 w590 w593 w596 w599 w602 w605 w608 w611 w614 w617] -> w49
                tunnel: [_ w85 w98 w99 w104 w105 w110 w129 _ _ w149 _ _ w162 _ _ w211 w219 w250 w251 _ w259 w270 w272 w277 w283 w288 w292 w295 w299 w302 _ w316 w319 w321 _ _ _ _ _ _ w398 w403 w406 w409 w412 w415 w424 _ w496 w499 w502 w505 w509 w510 w515 w520 w526 w529 w532 w535 w538 w541 w544 w547 w550 w553 w556 w559 w562 w565 w568 w571 w574 w577 w580 w583 w586 w589 w592 w595 w598 w601 w604 w607 w610 w613 w616] -> w43
                tunnel: [TRUE _ _ _ _ _ _ _ _ _ _ _ _ _ _ _ _ _ _ _ _ _ _ _ _ _ _ _ _ _ _ _ _ _ _ _ _ _ _ _ _ _ _ _ _ _ _ _ _ _ _ _ _ _ _ _ _ _ _ _ _ _ _ _ _ _ _ _ _ _ _ _ _ _ _ _ _ _ _ _ _ _ _ _ _ _ _ _] -> w45
                tunnel: w48 -> [w58 w86 w94 w101 w103 w106 w108 w127 w141 w145 w151 w154 w157 w161 w165 w189 w210 w218 w249 w252 w256 w258 w269 w273 w280 w282 w287 w291 w294 w298 w301 w311 w314 w317 w320 w323 w332 w362 w371 w384 w391 w397 w402 w405 w408 w411 w414 w423 w480 w495 w498 w501 w504 w508 w514 w519 w524 w525 w528 w531 w534 w537 w540 w543 w546 w549 w552 w555 w558 w561 w564 w567 w570 w573 w576 w579 w582 w585 w588 w591 w594 w597 w600 w603 w606 w609 w612 w615]
                tunnel: [w58 w87 w94 w101 w103 w106 w108 w127 w141 w145 w151 w154 w157 w161 w165 w189 w210 w218 w249 w252 w257 w258 w269 w273 w280 w282 w287 w291 w294 w298 w301 w311 w314 w317 w320 w323 w332 w362 w371 w384 w391 w397 w402 w405 w408 w411 w414 w423 w480 w495 w498 w501 w504 w508 w514 w519 w524 w525 w528 w531 w534 w537 w540 w543 w546 w549 w552 w555 w558 w561 w564 w567 w570 w573 w576 w579 w582 w585 w588 w591 w594 w597 w600 w603 w606 w609 w612 w615] -> w47
                tunnel: w40 -> [_ _ _ _ _ _ _ _ _ _ _ _ _ _ _ _ _ _ _ w253 _ _ _ _ _ _ _ _ _ _ _ _ _ _ _ _ _ _ _ _ _ _ _ _ _ _ _ _ _ _ _ _ _ _ _ _ _ _ _ _ _ _ _ _ _ _ _ _ _ _ _ _ _ _ _ _ _ _ _ _ _ _ _ _ _ _ _ _]
                event Timeout {
                  # "Update controls"
                  n9 = event-data() -> ()  [unwired: 1 in, 2 out]
                  n10 = Unbundle By Name(w78) -> ("Impulse Positions"=w81:T11, "No. Imp"=w79:i32, "Parameter Time Series"=w80:T2, "Parameter Impuls Series"=w82:T8, "Experiment Parameters.Freq"=w77:dbl, "Experiment Parameters.Vel"=w76:i32, "Experiment Parameters.Acc"=w75:i32, "Experiment Parameters.Stimulus"=w74:string, "Data File"=w73:T12, "desaccading parameters.Impulse Plane 2"=w71:T9, "desaccading parameters.Impulse dir"=w72:bool, "desacc.Threshold 1 [Acc]"=w70:dbl, "desacc.Threshold 2 [% of TH1]"=w63:i32, "desacc.tolerance"=w69:i32, "desacc.Search WD"=w61:dbl, "desacc.always use TH2"=w64:bool, "desacc.Range"=w68:dbl, "desacc.Max time"=w66:dbl, "desacc.Min time"=w65:dbl, "desacc.Velocity Threshold"=w57:i32, "filename"=w52:string, "calibration name"=w51:string)
                  n11 = local write "Freq."(w77) -> ()
                  n12 = local write "Vel."(w76) -> ()
                  n13 = local write "Acc"(w75) -> ()
                  n14 = Bundle("Max time"=w66, "Min time"=w65) -> (w67:cluster{"Max time":dbl, "Min time":dbl})  [unwired: 1 in]
                  n15 = local write "Impulse Positions"(w81) -> ()
                  n16 = local write "No. Imp"(w79) -> ()
                  n17 = local write "Parameter Time Series"(w80) -> ()
                  n18 = local write "Parameter Impuls Series"(w82) -> ()
                  n19 = local write "Stimulus type"(w74) -> ()
                  n20 = local write "Only Use TH-2"(w64) -> ()
                  n21 = local write "SD for Outlier detection"(w68) -> ()
                  n22 = local write "Velocity Threshold"(w57) -> ()
                  n23 = local write "Impulse dir"(w72) -> ()
                  n24 = local write "Threshold 2 [% of TH-1]"(w63) -> ()
                  n25 = local write "Tolerance [ms]"(w69) -> ()
                  n26 = local write "Impulse Plane 2"(w71) -> ()
                  n27 = local write "Accel Threshold [TH-1]"(w70) -> ()
                  n28 = local write "Saccade width [ms]"(w67) -> ()
                  n29 = local write "Data Output"(w73) -> ()
                  n30 = Unbundle By Name(w73) -> ("Channel List"=w56:string[])
                  n31 = Multiply(x=w61, y=1000.0 ("desacc .Search WD")) -> (x*y=w62:dbl)
                  n32 = local write "Search Window [ms]"(w62) -> ()
                  n33 = property on="Channel" class="Ring (strict)"("Strings []"=w56) -> ()  [unwired: 2 in, 2 out]
                  n34 = property on="Aligning Channel" class="Ring (strict)"("Strings []"=w56) -> ()  [unwired: 2 in, 2 out]
                  n35 = property on="Trigger Channel (Other)" class="Ring (strict)"("Strings []"=w56) -> ()  [unwired: 2 in, 2 out]
                  n36 = property on="List 1" class="Ring (strict)"("Strings []"=w56) -> ()  [unwired: 2 in, 2 out]
                  n37 = call <userlib>:"Current VIs Reference__ogtk.vi"() -> ("Current VI's reference"=w55:refnum<vi>)  [unwired: 5 in]
                  n38 = Concatenate Strings("EMA  -  " ("string"), w52) -> (w54:string)
                  n39 = local write "filename"(w52) -> ()
                  n40 = local write "calibration filename"(w51) -> ()
                  n41 = property class="VI"(reference=w55, "Front Panel.Title"=w54) -> ()  [unwired: 1 in, 2 out]
                }
                event User Event {
                  n42 = event-data() -> ("Double Click"=w84:path)  [unwired: 1 in, 3 out]
                  n43 = call <vilib>:"Get File Extension.vi"("file"=w84) -> ("lowercase file extension"=w83:string)  [unwired: 6 in, 4 out]
                  n44 = case shown="\"lvs\"" w83 {
                    tunnel: [w89 w91 w92 w93] -> w85
                    frame "hrch" {
